vi "CTL_Fill-DrainJog.vi"(7 "Pump CtlRef In":T3, 11 "Pump Cmds":T1) -> (1 "Drain Out":bool, 2 "Fill Out":bool, 3 "Err":bool, 5 "Run Btn":bool)   [LabVIEW 2024]
doc: "Input is reference to front panel buttons Cluster. Excludes Fill and Drain buttons from being activated at the same time. \nIf Jog is FALSE then Fill or Drain Cmd states provided by some remote controller are output. \nelse Fill and Drain button states are output\nThe current output state is indicated on the front panel buttons."
uses:
  Control Definitions/Def PumpCtlRefs.ctl
  Control Definitions/Def_PumpSpeed.ctl
  Control Definitions/Def_PumpCmds.ctl
panel:
  out "Pump Speed Out":enum16{"FAST", "SLOW", "CREEP", "STOP"}(ring)
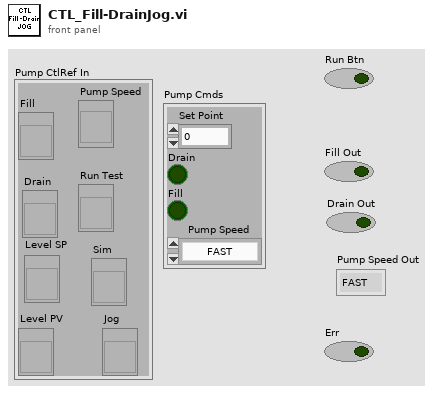
[diagram p1: front panel]
types:
  T1 = typedef "Def_PumpCmds.ctl" = cluster{"Set Point":dbl, "Drain":bool, "Fill":bool, "Pump Speed ":T2}
  T2 = typedef "Def_PumpSpeed.ctl" = enum16{"FAST", "SLOW", "CREEP", "STOP"}
  T3 = typedef "Def PumpCtlRefs.ctl" = cluster{"Fill ":refnum<vi>, "Drain":refnum<vi>, "Level PV":refnum<vi>, "Pump Speed":refnum<vi>, "Run Test":refnum<vi>, "Sim":refnum<vi>, "Jog":refnum<vi>, "Level SP":refnum<vi>}
  T4 = enum8{"Enabled", "Disabled", "Disabled and Grayed Out"}
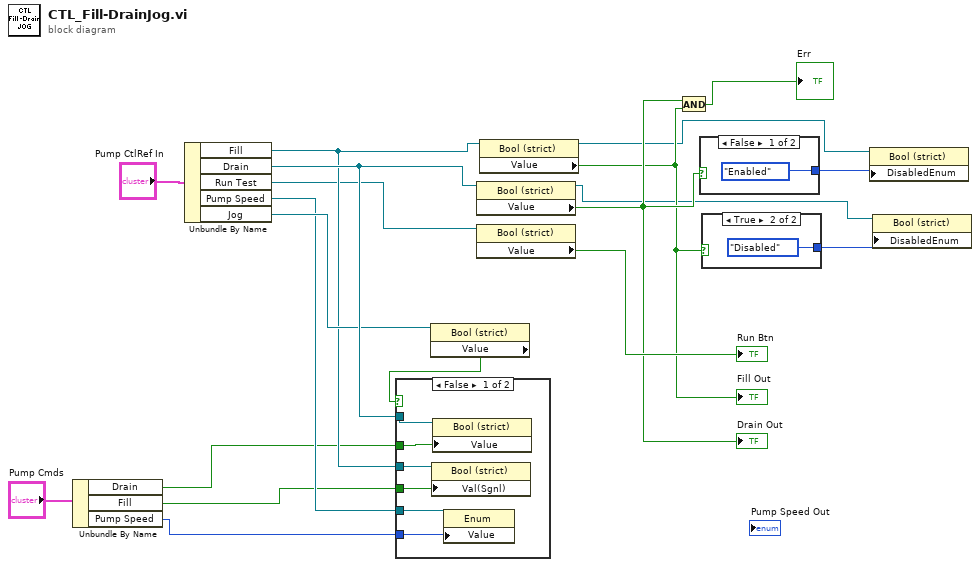
[diagram p0: block diagram]
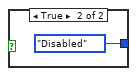
[diagram p3: hidden frame]
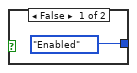
[diagram p4: hidden frame]
diagram:
  n1 = Unbundle By Name("Pump Cmds") -> ("Drain"=w2:bool, "Fill"=w3:bool, "Pump Speed"=w1:T2)
  n2 = Unbundle By Name("Pump CtlRef In") -> ("Fill"=w7:refnum<vi>, "Drain"=w17:refnum<vi>, "Run Test"=w6:refnum<vi>, "Pump Speed"=w5:refnum<vi>, "Jog"=w9:refnum<vi>)
  n3 = property on="Property Node" class="Bool (strict)"(reference=w9) -> ("Value"=w8:bool)  [unwired: 1 in, 2 out]
  n4 = case shown="False" w8 {
    tunnel: w3 -> [w25 _]
    tunnel: w7 -> [w24 _]
    tunnel: w2 -> [w23 _]
    tunnel: w17 -> [w22 _]
    tunnel: w1 -> [w20 _]
    tunnel: w5 -> [w21 _]
    frame False {
      n5 = property class="Bool (strict)"(reference=w24, "Val(Sgnl)"=w25) -> ()  [unwired: 1 in, 2 out]
      n6 = property class="Bool (strict)"(reference=w22, "Value"=w23) -> ()  [unwired: 1 in, 2 out]
      n7 = property class="Enum"(reference=w21, "Value"=w20) -> ()  [unwired: 1 in, 2 out]
    }
    frame True {
    }
  }
  n8 = property on="Property Node" class="Bool (strict)"(reference=w17) -> (reference out=w14:refnum<vi>, "Value"=w16:bool)  [unwired: 1 in, 1 out]
  "Drain Out" <- w16
  n9 = property on="Property Node" class="Bool (strict)"(reference=w6) -> ("Value"=→"Run Btn":bool)  [unwired: 1 in, 2 out]
  n10 = property on="Property Node" class="Bool (strict)"(reference=w7) -> (reference out=w13:refnum<vi>, "Value"=w15:bool)  [unwired: 1 in, 1 out]
  "Fill Out" <- w15
  n11 = And(x=w16, y=w15) -> (x .and. y?=→"Err":bool)
  n12 = case shown="False" w16 {
    tunnel: [T4."Enabled" ("Disabled") T4."Disabled" ("Disabled")] -> w11
    frame False {
    }
    frame True {
    }
  }
  n13 = case shown="True" w15 {
    tunnel: [T4."Enabled" ("Disabled") T4."Disabled" ("Disabled")] -> w12
    frame False {
    }
    frame True {
    }
  }
  n14 = property on="Property Node" class="Bool (strict)"(reference=w13, "DisabledEnum"=w11) -> ()  [unwired: 1 in, 2 out]
  n15 = property on="Property Node" class="Bool (strict)"(reference=w14, "DisabledEnum"=w12) -> ()  [unwired: 1 in, 2 out]
